vi "FTW-JSON-Object-Update.vi"(0 "JSON Object":refnum<data-value>, 5 "JSON Object to Merge":string, 7 "Update Mode":T1, 11 "error in":errorcluster) -> (4 "JSON Object out":refnum<data-value>, 15 "error out":errorcluster)   [LabVIEW 2015]
uses:
  core/FTW-JSON-Core-Structure.ctl
  FTW-JSON-UpdateMode.ctl
panel:
  # "Inputs"
  # "Outputs"
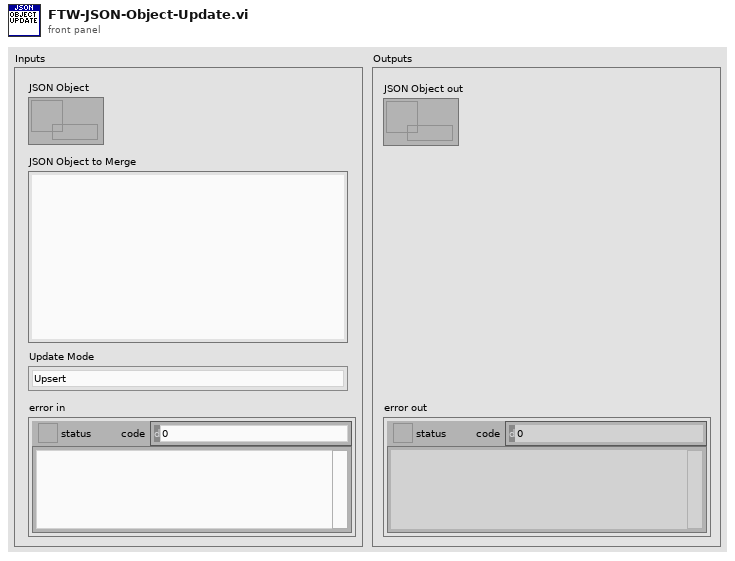
[diagram p1: front panel]
types:
  T1 = typedef "FTW-JSON-UpdateMode.ctl" = enum32{"Upsert", "Update Only", "Insert Only"}
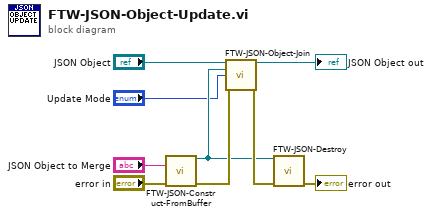
[diagram p0: block diagram]
diagram:
  n1 = call "FTW-JSON-Construct-FromBuffer.vi"("JSON String (UTF-8)"="JSON Object to Merge", "error in"="error in") -> ("JSON Object"=w2:refnum<data-value>, "error out"=w4:errorcluster)  [unwired: 12 in]
  n2 = call "FTW-JSON-Object-Join.vi"("JSON Object"="JSON Object", "JSON Object to Merge"=w2, "Join Mode"="Update Mode", "error in"=w4) -> ("JSON Object out"=→"JSON Object out":refnum<data-value>, "error out"=w3:errorcluster)  [unwired: 10 in]
  n3 = call "FTW-JSON-Destroy.vi"("JSON Object"=w2, "error in"=w3) -> ("error out"=→"error out":errorcluster)  [unwired: 13 in]
